vi "Convert to String_I8.vi"(4 "Input":dbl) -> (1 "String (I8)":string)   [LabVIEW 2012]
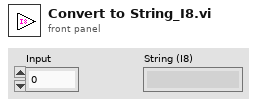
[diagram p1: front panel]
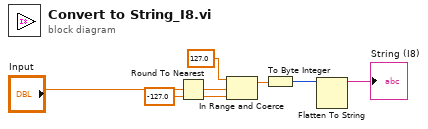
[diagram p0: block diagram]
diagram:
  n1 = Round To Nearest(number="Input") -> (nearest integer value=w1:dbl)
  n2 = In Range and Coerce(upper limit=127.0, x=w1, lower limit=-127.0 ("upper limit")) -> (coerced(x)=w4:dbl)  [unwired: 1 out]
  n3 = To Byte Integer(number=w4) -> (8bit integer=w5:i8)
  n4 = Flatten To String(anything=w5) -> (data string=→"String (I8)":string)  [unwired: 3 in, 2 out]
